vi "Set Optimiser Cell.vi"(8 "error in (no error)":errorcluster, 10 "Schedule Cell":refnum<class "Optimiser Cell.lvclass">, 11 "Optimiser SBlock in":refnum<class "Optimiser SBlock.lvclass">) -> (0 "error out":errorcluster, 3 "Optimiser SBlock out":refnum<class "Optimiser SBlock.lvclass">)   [LabVIEW 2020, in "Run Utilities.lvlib" / "Optimiser SBlock.lvclass"]
uses:
  Optimiser SBlock.lvclass
  C:/Users/marco/Documents/GitHub_Lab/TALOS/talos/Run Utilities/Schedule Block/Schedule Block.lvclass
  Optimiser Cell/Optimiser Cell.lvclass
  C:/Users/marco/Documents/GitHub_Lab/TALOS/talos/Run Utilities/Cell/Schedule Cell.lvclass
  Schedule/Schedule.lvclass
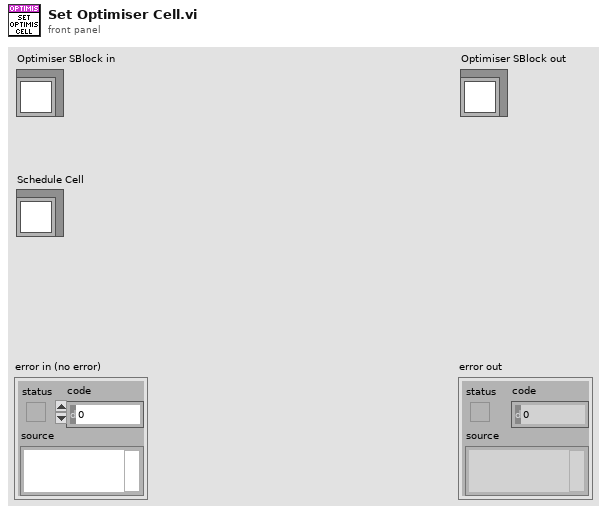
[diagram p1: front panel]
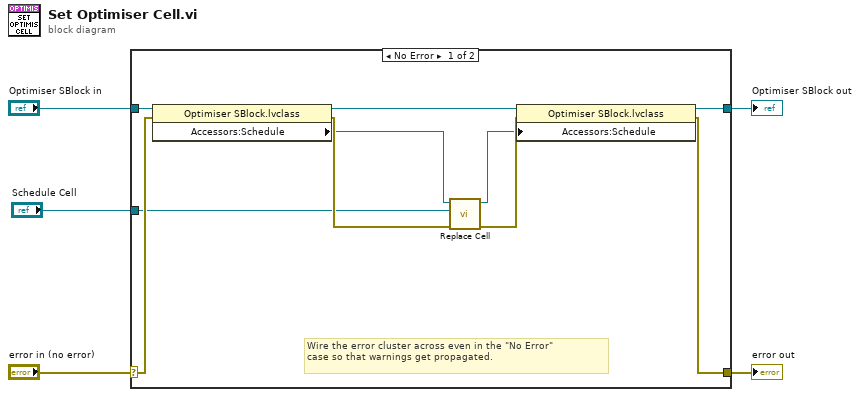
[diagram p0: block diagram]
diagram:
  n1 = case shown="No Error" "error in (no error)" {
    selector: "error in (no error)" -> [w15 w17]
    tunnel: [w12 w17] -> w4
    tunnel: [w10 w16] -> w2
    tunnel: "Optimiser SBlock in" -> [w11 w16]
    tunnel: "Schedule Cell" -> [w6 _]
    frame No Error {
      # "Wire the error cluster across even in the \"No Error\"\ncase so that warnings get propagated."
      n2 = property class="Optimiser SBlock.lvclass"(reference=w11, error in=w15) -> (reference out=w9:refnum<class "Optimiser SBlock.lvclass">, error out=w14:errorcluster, "Accessors:Schedule"=w7:refnum<class "Schedule.lvclass">)
      n3 = call-dynamic "Replace Cell.vi"("error in (no error)"=w14, "Schedule Cell"=w6, "Schedule in"=w7) -> ("error out"=w13:errorcluster, "Schedule out"=w8:refnum<class "Schedule.lvclass">)  [unwired: 7 in]
      n4 = property class="Optimiser SBlock.lvclass"(reference=w9, error in=w13, "Accessors:Schedule"=w8) -> (reference out=w10:refnum<class "Optimiser SBlock.lvclass">, error out=w12:errorcluster)
    }
    frame Error {
    }
  }
  "error out" <- w4
  "Optimiser SBlock out" <- w2
